vi "Periodic Tasks.vi"(8 "error in":errorcluster) -> ()   [LabVIEW 2017]
doc: "This VI runs in parallel to other tasks. It can contain as many user-defined periodic loops as you need. These can carry out PID or other sorts of timed response."
uses:
  <vilib>/Rock Robotics/WPI/Utilities/WPI_GetSetVariantRefNum.vi
panel:
  out "Estado":dbl
  out "Valor Motor":dbl
  in  "Segurando":dbl
  in  "Expelir":dbl
  in  "Coletar":dbl
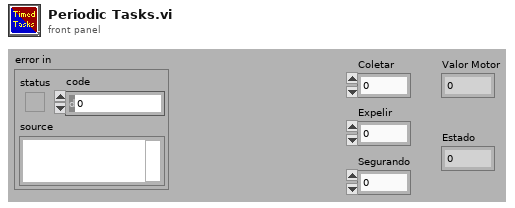
[diagram p1: front panel]
types:
  T1 = enum16{"Repouso", "Coletar", "Segurando", "Expelindo"}
  T2 = typedef "WPI_JoystickDevRef.ctl" = cluster{"Device":T3}
  T3 = typedef "WPI_JoystickDeviceEnum.ctl" = enum16{"USB 0", "USB 1", "USB 2", "USB 3", "USB 4", "USB 5"}
  T4 = cluster{"Buttons[0]":bool, "Buttons[1]":bool, "Buttons[2]":bool, "Buttons[3]":bool, "Buttons[4]":bool, "Buttons[5]":bool, "Buttons[6]":bool, "Buttons[7]":bool, "Buttons[8]":bool}
  T5 = typedef "WPI_MotorControlDeviceRef.ctl" = cluster{"DeviceStatus":errorcluster, "Type":T6, "PWM":cluster{"PWM Channel":T7, "DeadBand":T8}, "CAN":cluster{"Device Number":u8, "SetOutput VI Ref":variant, "GetOutput VI Ref":variant, "Enable VI Ref":variant, "Disable VI Ref":variant, "Data":variant}, "Invert":bool, "DIO PWM":cluster{"PWM \"Enable\" Channel":T7, "DIOChannel":T9, "PWM Rate":dbl}}
  T6 = typedef "WPI_MotorControlType.ctl" = enum16{"PWM", "CAN", "DIO PWM"}
  T7 = typedef "FPGA_DIOPWMChannel.ctl" = enum8{"PWM 0", "PWM 1", "PWM 2", "PWM 3", "PWM 4", "PWM 5", "PWM 6", "PWM 7", "PWM 8", "PWM 9", "PWM MXP 0", "PWM MXP 1", "PWM MXP 2", "PWM MXP 3", "PWM MXP 4", "PWM MXP 5", "PWM MXP 6", "PWM MXP 7", "PWM MXP 8", "PWM MXP 9", "Invalid"}
  T8 = typedef "WPI_PWMDeadband.ctl" = cluster{"Name":string, "maxPositivePwm":i32, "minPositivePwm":i32, "centerPwm":i32, "maxNegativePwm":i32, "minNegativePwm":i32, "angularRange":u16}
  T9 = typedef "FPGA_DIOChannel.ctl" = enum8{"DIO 0", "DIO 1", "DIO 2", "DIO 3", "DIO 4", "DIO 5", "DIO 6", "DIO 7", "DIO 8", "DIO 9", "DIO MXP 0", "DIO MXP 1", "DIO MXP 2", "DIO MXP 3", "DIO MXP 4", "DIO MXP 5", "DIO MXP 6", "DIO MXP 7", "DIO MXP 8", "DIO MXP 9", "DIO MXP 10", "DIO MXP 11", "DIO MXP 12", "DIO MXP 13", "DIO MXP 14", "DIO MXP 15", "SPI Port CS1", "SPI Port CS2", "SPI Port CS3", "SPI Port MISO", "SPI Port MOSI", "Invalid"}
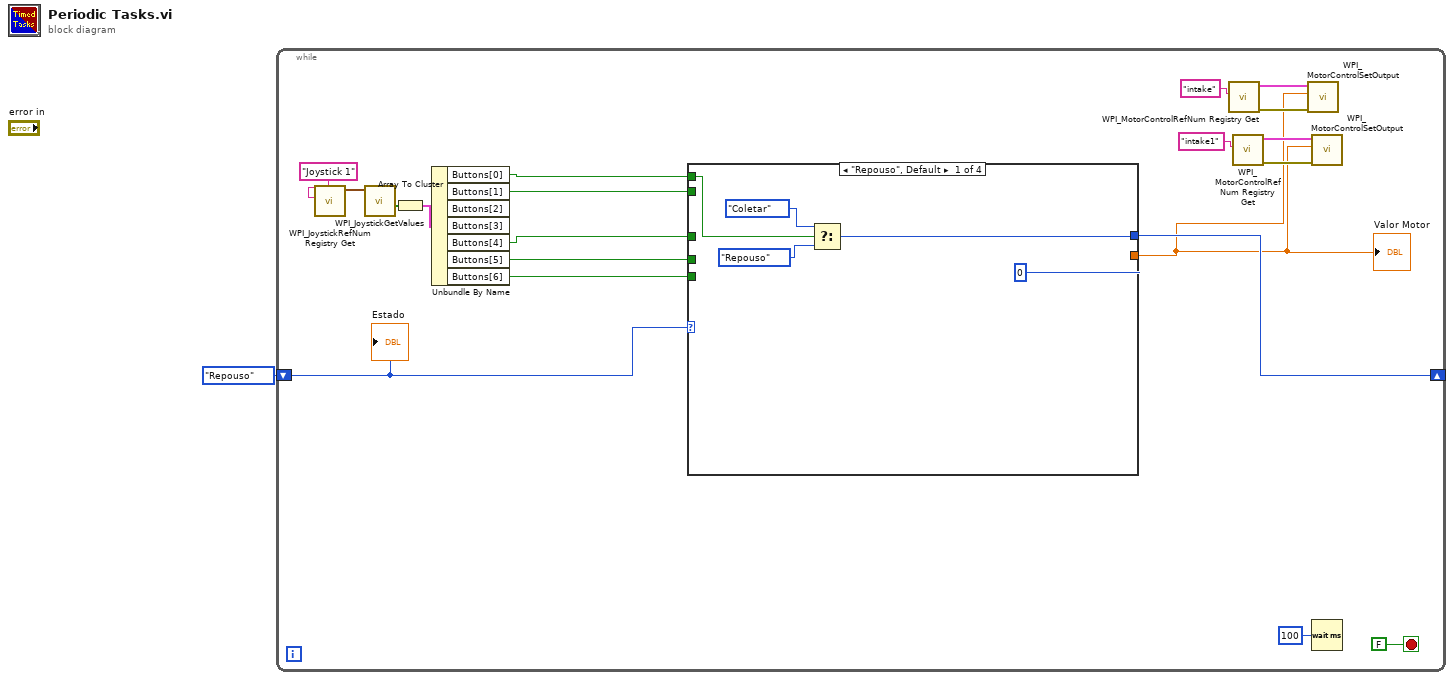
[diagram p0: block diagram]
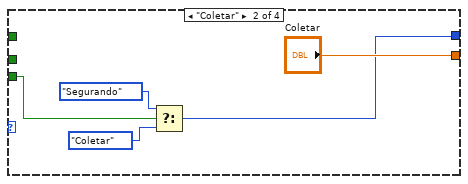
[diagram p2: hidden frame]
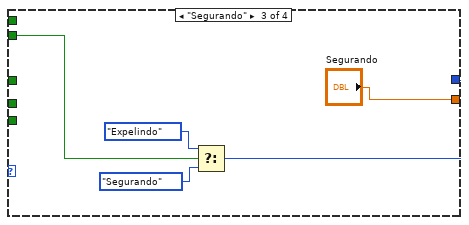
[diagram p3: hidden frame]
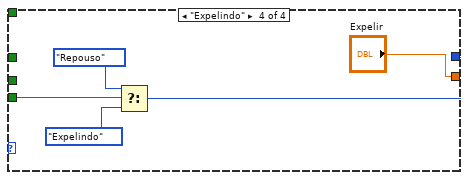
[diagram p4: hidden frame]
diagram:
  n1 = while {
    shift-right: [w19] -> _
    shift-left: T1."Repouso" -> [w18]
    stop <- FALSE stop-if-true
    n2 = call <vilib>:"WPI_JoystickRefNum Registry Get.vi"("refnum name"="Joystick 1") -> ("JoystickDevRef"=w8:T2)  [unwired: 1 in, 9 out]
    n3 = call <vilib>:"WPI_JoystickGetValues.vi"("JoystickDevRef"=w8) -> ("Buttons"=w9:bool[])  [unwired: 6 in, 4 out]
    n4 = Array To Cluster(array=w9) -> (cluster=w10:T4)
    n5 = Unbundle By Name(w10) -> ("Buttons[0]"=w6:bool, "Buttons[1]"=w5:bool, "Buttons[4]"=w3:bool, "Buttons[5]"=w2:bool, "Buttons[6]"=w4:bool)  [unwired: 2 out]
    n6 = case shown="\"Repouso\", Default" w18 {
      tunnel: w6 -> [w22 _ _ _]
      tunnel: [w24 w29 w32 w39] -> w19
      tunnel: [0 "Coletar" "Segurando" "Expelir"] -> w13
      tunnel: w5 -> [_ _ w35 _]
      tunnel: w4 -> [_ w27 _ w37]
      tunnel: w3 -> [_ _ _ _]
      tunnel: w2 -> [_ _ _ _]
      frame "Repouso", Default {
        n7 = Select(t=T1."Coletar", s=w22, f=T1."Repouso") -> (s? t:f=w24:T1)
      }
      frame "Coletar" {
        n8 = Select(t=T1."Segurando", s=w27, f=T1."Coletar") -> (s? t:f=w29:T1)
      }
      frame "Segurando" {
        n9 = Select(t=T1."Expelindo", s=w35, f=T1."Segurando") -> (s? t:f=w32:T1)
      }
      frame "Expelindo" {
        n10 = Select(t=T1."Repouso", s=w37, f=T1."Expelindo") -> (s? t:f=w39:T1)
      }
    }
    "Valor Motor" <- w13
    n11 = call <vilib>:"WPI_MotorControlRefNum Registry Get.vi"("refnum name"="intake") -> ("error out"=w15:errorcluster, "MotorControlDevRef"=w14:T5)  [unwired: 9 in]
    n12 = call <vilib>:"WPI_MotorControlRefNum Registry Get.vi"("refnum name"="intake1") -> ("error out"=w17:errorcluster, "MotorControlDevRef"=w16:T5)  [unwired: 9 in]
    n13 = call <vilib>:"WPI_MotorControlSetOutput.vi"("error in (no error)"=w15, "Output"=w13, "MotorControlDevRef"=w14) -> ()  [unwired: 6 in, 3 out]
    n14 = call <vilib>:"WPI_MotorControlSetOutput.vi"("error in (no error)"=w17, "Output"=w13, "MotorControlDevRef"=w16) -> ()  [unwired: 6 in, 3 out]
    n15 = Wait (ms)(milliseconds to wait=u32 100) -> ()  [unwired: 1 out]
    "Estado" <- w18
  }
